vi "ConnectCaseStructureTunnel__slk_mt.vi"(8 "error in (no error)":errorcluster, 10 "case structure refnum in":refnum<vi>, 11 "diagram refnum in":refnum<vi>) -> (0 "error out":errorcluster, 2 "duplicated case structure refnum out":refnum<vi>, 3 "duplicated diagram refnum out":refnum<vi>)   [LabVIEW 2012, in "Lazyboots Menu Tool.lvlib"]
doc: "Connects error selector/tunnel of error case."
uses:
  Library/Lazyboots Menu Tool.lvlib
  TypeDef/TypeDef_ConnectCaseStructureTunnelState__slk_mt.ctl
panel:
  # "ConnectCaseStructureTunnel__slk_mt.vi\nConnects error selector/tunnel of error case.\n\nNOTICE -- YOU MUST LEAVE THIS NOTICE IN PLACE.\n\nCopyright (c) 2011, LIANG LIU Shawn.Liu.cn@gmail.com\nAll rights reserved.\n\nRedistribution and use in source and binary forms, with or without modification, are permitted provided that the following conditions are met:\n-Redistributions of source code must retain the above copyright notice, this list of conditions and the following disclaimer.\n-Redistributions in binary form must reproduce the above copyright notice, this list of conditions and the following disclaimer in the documentation and/or other materials provided with the distribution.\n-Neither the name of the eLp nor the names of its contributors may be used to endorse or promote products derived from this software without specific prior written permission.\n\nTHIS SOFTWARE IS PROVIDED BY THE COPYRIGHT HOLDERS AND CONTRIBUTORS \"AS IS\" AND ANY EXPRESS OR IMPLIED WARRANTIES, INCLUDING, BUT NOT LIMITED TO, THE IMPLIED WARRANTIES OF MERCHANTABILITY AND FITNESS FOR A PARTICULAR PURPOSE ARE DISCLAIMED. IN NO EVENT SHALL THE COPYRIGHT HOLDER OR CONTRIBUTORS BE LIABLE FOR ANY DIRECT, INDIRECT, INCIDENTAL, SPECIAL, EXEMPLARY, OR CONSEQUENTIAL DAMAGES (INCLUDING, BUT NOT LIMITED TO, PROCUREMENT OF SUBSTITUTE GOODS OR SERVICES; LOSS OF USE, DATA, OR PROFITS; OR BUSINESS INTERRUPTION) HOWEVER CAUSED AND ON ANY THEORY OF LIABILITY, WHETHER IN CONTRACT, STRICT LIABILITY, OR TORT (INCLUDING NEGLIGENCE OR OTHERWISE) ARISING IN ANY WAY OUT OF THE USE OF THIS SOFTWARE, EVEN IF ADVISED OF THE POSSIBILITY OF SUCH DAMAGE."
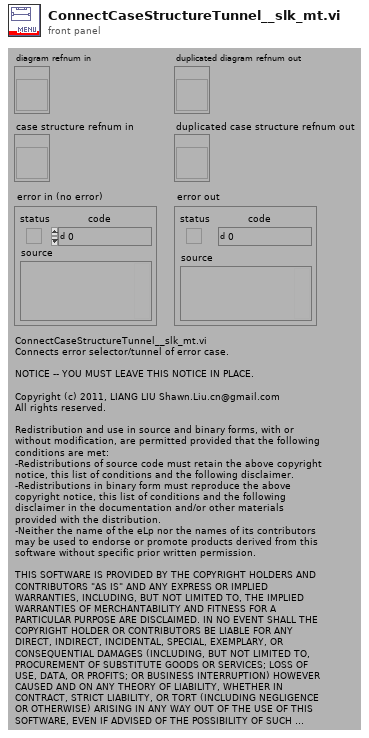
[diagram p1: front panel]
types:
  T1 = typedef "Lazyboots Menu Tool.lvlib/TypeDef_ConnectCaseStructureTunnelState__slk_mt.ctl" = enum16{"Get error in/out tunnel", "No Error.Connect selector outside", "No Error.Connect selector inside", "No Error.Move selector", "Show error case", "Error.Connect selector inside", "Show no error case", "End"}
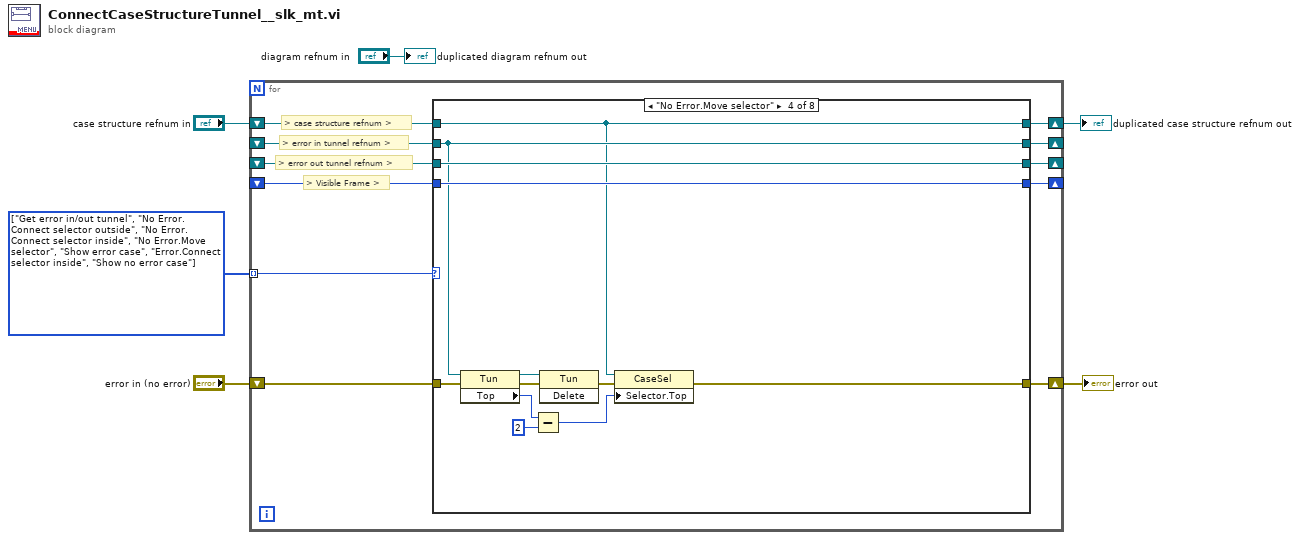
[diagram p0: block diagram]
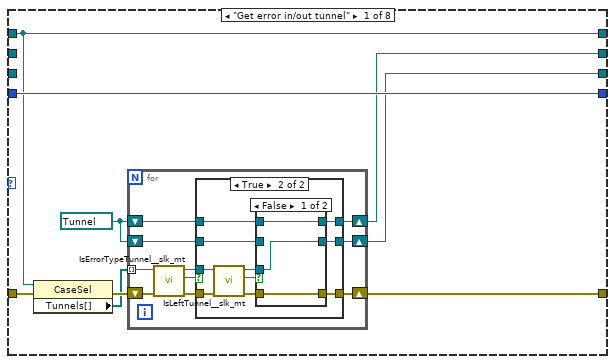
[diagram p2: hidden frame]
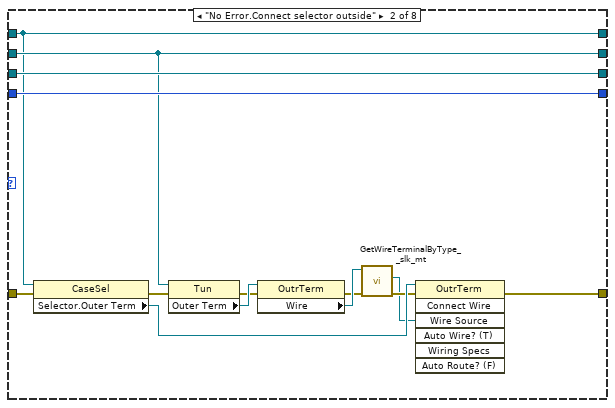
[diagram p5: hidden frame]
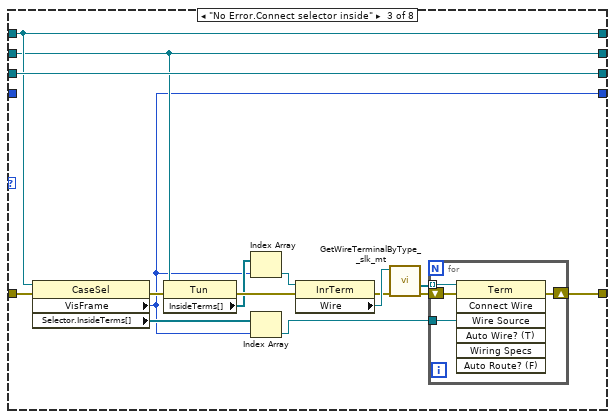
[diagram p6: hidden frame]
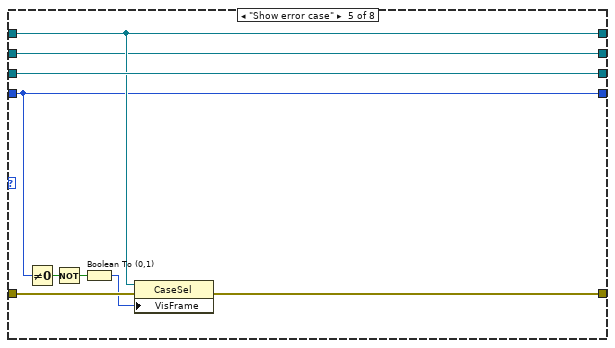
[diagram p7: hidden frame]
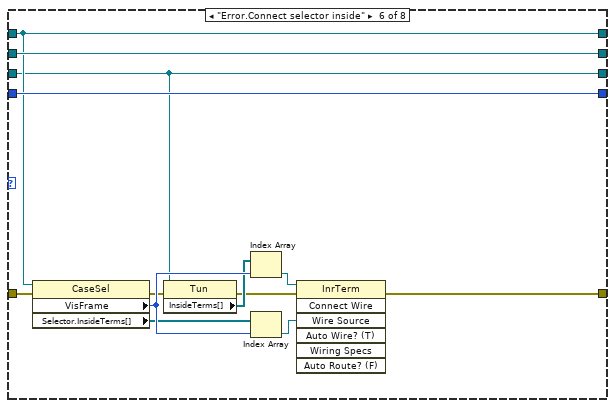
[diagram p8: hidden frame]
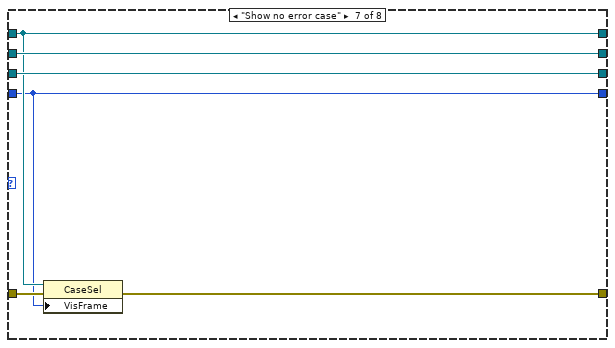
[diagram p9: hidden frame]
diagram:
  w2 = T1[] [enum."Get error in/out tunnel", enum."No Error.Connect selector outside", enum."No Error.Connect selector inside", enum."No Error.Move selector", enum."Show error case", enum."Error.Connect selector inside", enum."Show no error case"] items=["Get error in/out tunnel", "No Error.Connect selector outside", "No Error.Connect selector inside", "No Error.Move selector", "Show error case", "Error.Connect selector inside", "Show no error case", "End"]
  n1 = for {
    shift-right: [w16] -> w4
    shift-left: "case structure refnum in" -> [w17]
    shift-right: [w10] -> _
    shift-left: _ -> [w15]
    shift-right: [w11] -> _
    shift-left: _ -> [w14]
    shift-right: [w12] -> _
    shift-left: _ -> [w13]
    shift-right: [w8] -> w1
    shift-left: "error in (no error)" -> [w9]
    tunnel: w2 -> [w7] mode=indexing
    # "> Visible Frame >"
    # "> error out tunnel refnum >"
    # "> case structure refnum >"
    # "> error in tunnel refnum >"
    n2 = case shown="\"No Error.Move selector\"" w7 {
      tunnel: w17 -> [w23 w56 w73 w93 w109 w113 w125 w132]
      tunnel: [w23 w56 w73 w93 w109 w113 w125 w132] -> w16
      tunnel: w15 -> [_ w57 w72 w96 w108 w123 w129 w134]
      tunnel: w14 -> [_ w68 w85 w100 w110 w112 w128 w133]
      tunnel: w13 -> [w26 w69 _ w101 w104 w122 w124 w131]
      tunnel: [w26 w69 w70 w101 w104 w122 w124 w131] -> w12
      tunnel: [w19 w68 w85 w100 w110 w112 w128 w133] -> w11
      tunnel: [w20 w57 w72 w96 w108 w123 w129 w134] -> w10
      tunnel: w9 -> [w25 w59 w74 w91 w106 w114 w127 w130]
      tunnel: [w18 w58 w71 w95 w107 w111 w126 w130] -> w8
      frame "Get error in/out tunnel" {
        w21 = refnum<vi> refnum ("reference out")
        n3 = property class="CaseSel"(reference=w23, error in=w25) -> (error out=w24:errorcluster, "Tunnels[]"=w22:refnum<vi>[])  [unwired: 1 out]
        n4 = for {
          shift-right: [w29] -> w20
          shift-left: w21 -> [w31]
          tunnel: w22 -> [w35] mode=indexing
          shift-right: [w28] -> w19
          shift-left: w21 -> [w30]
          shift-right: [w27] -> w18
          shift-left: w24 -> [w36]
          n5 = call "IsErrorTypeTunnel__slk_mt.vi"("error in (no error)"=w36, "tunnel refnum in"=w35) -> ("error out"=w33:errorcluster, "error type tunnel?"=w32:bool, "duplicated tunnel refnum out"=w34:refnum<vi>)  [unwired: 7 in]
          n6 = case shown="True" w32 {
            tunnel: w34 -> [_ w49]
            tunnel: w33 -> [w37 w48]
            tunnel: w31 -> [w39 w44]
            tunnel: w30 -> [w38 w43]
            tunnel: [w39 w41] -> w29
            tunnel: [w38 w42] -> w28
            tunnel: [w37 w40] -> w27
            frame False {
            }
            frame True {
              n7 = call "IsLeftTunnel__slk_mt.vi"("error in (no error)"=w48, "tunnel refnum in"=w49) -> ("error out"=w46:errorcluster, "left tunnel?"=w47:bool, "duplicated tunnel refnum out"=w45:refnum<vi>)  [unwired: 7 in]
              n8 = case shown="False" w47 {
                tunnel: w46 -> [w50 w53]
                tunnel: w45 -> [w52 w54]
                tunnel: w44 -> [w51 _]
                tunnel: w43 -> [_ w55]
                tunnel: [w52 w55] -> w42
                tunnel: [w51 w54] -> w41
                tunnel: [w50 w53] -> w40
                frame False {
                }
                frame True {
                }
              }
            }
          }
        }
      }
      frame "No Error.Connect selector outside" {
        n9 = property class="CaseSel"(reference=w56, error in=w59) -> (error out=w66:errorcluster, "Selector.Outer Term"=w67:refnum<vi>)  [unwired: 1 out]
        n10 = property class="Tun"(reference=w57, error in=w66) -> (error out=w63:errorcluster, "Outer Term"=w65:refnum<vi>)  [unwired: 1 out]
        n11 = property class="OutrTerm"(reference=w65, error in=w63) -> (error out=w62:errorcluster, "Wire"=w64:refnum<vi>)  [unwired: 1 out]
        n12 = call "GetWireTerminalByType__slk_mt.vi"("error in (no error)"=w62, "wire refnum in"=w64) -> ("error out"=w61:errorcluster, "source terminal out"=w60:refnum<vi>)  [unwired: 8 out]
        n13 = invoke class="OutrTerm" method="Connect Wire"(reference=w67, error in=w61, "Wire Source"=w60) -> (error out=w58:errorcluster)  [unwired: 4 in, 6 out]
      }
      frame "No Error.Connect selector inside" {
        n14 = property class="CaseSel"(reference=w73, error in=w74) -> (error out=w83:errorcluster, "VisFrame"=w70:u32, "Selector.InsideTerms[]"=w84:refnum<vi>[])  [unwired: 1 out]
        n15 = property class="Tun"(reference=w72, error in=w83) -> (error out=w82:errorcluster, "InsideTerms[]"=w81:refnum<vi>[])  [unwired: 1 out]
        n16 = Index Array(array=w81, index=w70) -> (element=w80:refnum<vi>)
        n17 = Index Array(array=w84, index=w70) -> (element=w79:refnum<vi>)
        n18 = property class="InrTerm"(reference=w80, error in=w82) -> (error out=w75:errorcluster, "Wire"=w76:refnum<vi>)  [unwired: 1 out]
        n19 = call "GetWireTerminalByType__slk_mt.vi"("error in (no error)"=w75, "wire refnum in"=w76) -> ("error out"=w77:errorcluster, "sink terminals out"=w78:refnum<vi>[])  [unwired: 8 out]
        n20 = for {
          tunnel: w78 -> [w89] mode=indexing
          shift-right: [w87] -> w71
          shift-left: w77 -> [w88]
          tunnel: w79 -> [w86]
          n21 = invoke class="Term" method="Connect Wire"(reference=w89, error in=w88, "Wire Source"=w86) -> (error out=w87:errorcluster)  [unwired: 4 in, 6 out]
        }
      }
      frame "No Error.Move selector" {
        n22 = property class="Tun"(reference=w96, error in=w91) -> (reference out=w99:refnum<vi>, error out=w98:errorcluster, "Top"=w92:i32)
        n23 = Subtract(x=w92, y=2) -> (x-y=w94:i32)
        n24 = invoke class="Tun" method="Delete"(reference=w99, error in=w98) -> (error out=w97:errorcluster)  [unwired: 1 in, 2 out]
        n25 = property class="CaseSel"(reference=w93, error in=w97, "Selector.Top"=w94) -> (error out=w95:errorcluster)  [unwired: 1 out]
      }
      frame "Show error case" {
        n26 = Not Equal To 0?(x=w104) -> (x != 0?=w105:bool)
        n27 = Not(x=w105) -> (.not. x?=w103:bool)
        n28 = Boolean To (0,1)(Boolean=w103) -> (0, 1=w102:i16)
        n29 = property class="CaseSel"(reference=w109, error in=w106, "VisFrame"=w102) -> (error out=w107:errorcluster)  [unwired: 1 out]
      }
      frame "Error.Connect selector inside" {
        n30 = property class="CaseSel"(reference=w113, error in=w114) -> (error out=w117:errorcluster, "VisFrame"=w121:u32, "Selector.InsideTerms[]"=w116:refnum<vi>[])  [unwired: 1 out]
        n31 = property class="Tun"(reference=w112, error in=w117) -> (error out=w118:errorcluster, "InsideTerms[]"=w120:refnum<vi>[])  [unwired: 1 out]
        n32 = Index Array(array=w120, index=w121) -> (element=w119:refnum<vi>)
        n33 = Index Array(array=w116, index=w121) -> (element=w115:refnum<vi>)
        n34 = invoke class="InrTerm" method="Connect Wire"(reference=w119, error in=w118, "Wire Source"=w115) -> (error out=w111:errorcluster)  [unwired: 4 in, 6 out]
      }
      frame "Show no error case" {
        n35 = property class="CaseSel"(reference=w125, error in=w127, "VisFrame"=w124) -> (error out=w126:errorcluster)  [unwired: 1 out]
      }
      frame "End" {
      }
    }
  }
  "duplicated case structure refnum out" <- w4
  "error out" <- w1
  "duplicated diagram refnum out" <- "diagram refnum in"
